vi "2L06-lambda_1D_n1.vi"(0 "OBS/MIF":enum16{"OBS", "MIF"}(ring), 7 "t":dbl[](array[numeric]), 9 "N(t)":u32[](array[numeric]), 11 "error in":errorcluster) -> (4 "Lambda":dbl[](array[numeric]), 15 "error out":errorcluster)   [LabVIEW 2010, in "lv_02.lvlib"]
doc: "Calcul du taux de défaillance à partir de la série t et de la série des effectifs encore en fonctionnement à t :\nObs : précise si les observations sont fournies par rang (n obs) ou par classe (nc classes)\nSi N(t=0) est nul ou non câblé pour les observations de type obs_n, alors n= taille du tableau t"
uses:
  lv_02.lvlib
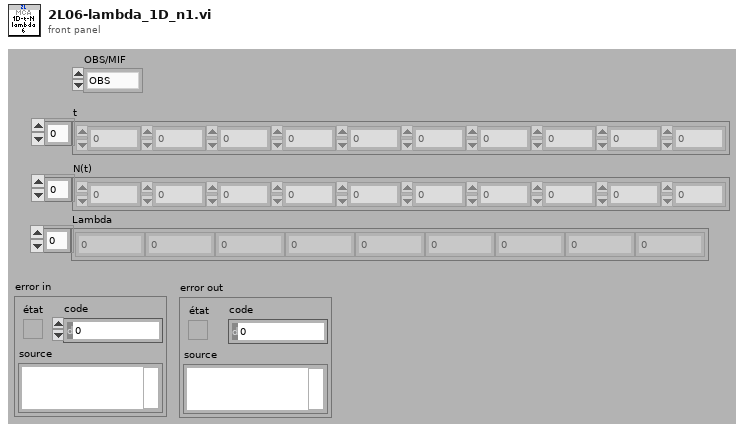
[diagram p1: front panel]
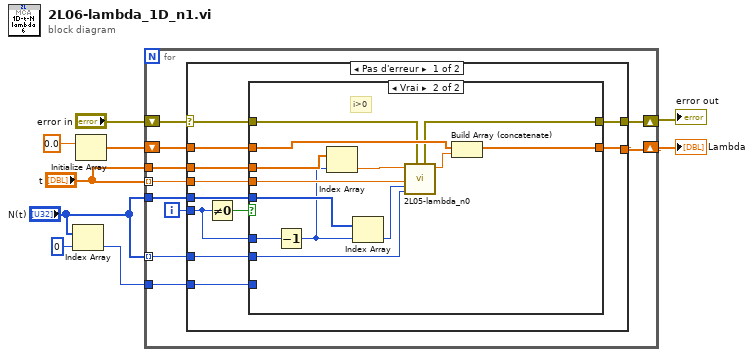
[diagram p0: block diagram]
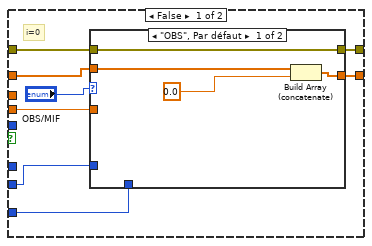
[diagram p2: hidden frame]
diagram:
  n1 = Index Array(array="N(t)", index=0 ("indice")) -> (element=w1:u32)
  n2 = Initialize Array(0.0 ("élément")) -> (w6:dbl[])  [unwired: 1 in]
  n3 = for {
    tunnel: "t" -> [w17]
    tunnel: "t" -> [w19] mode=indexing
    tunnel: "N(t)" -> [w18] mode=indexing
    tunnel: "N(t)" -> [w16]
    shift-right: [w14] -> w4
    shift-left: w6 -> [w15]
    shift-right: [w13] -> w5
    shift-left: "error in" -> [w12]
    tunnel: w1 -> [w10]
    i -> [w11]
    n4 = case shown="Pas d'erreur" w12 {
      selector: w12 -> [w25 w59]
      tunnel: w19 -> [w22 _]
      tunnel: w18 -> [w30 _]
      tunnel: w17 -> [w23 _]
      tunnel: w16 -> [w29 _]
      tunnel: w15 -> [w28 w58]
      tunnel: [w27 w58] -> w14
      tunnel: [w26 w59] -> w13
      tunnel: w11 -> [w21 _]
      tunnel: w10 -> [w20 _]
      frame No Error {
        n5 = Not Equal To 0?(x=w21) -> (x != 0?=w24:bool)
        n6 = case shown="Vrai" w24 {
          tunnel: w29 -> [_ w57]
          tunnel: [w34 w50] -> w27
          tunnel: w30 -> [w38 w56]
          tunnel: w23 -> [_ w55]
          tunnel: w28 -> [w35 w52]
          tunnel: [w33 w49] -> w26
          tunnel: w25 -> [w37 w48]
          tunnel: w22 -> [w36 w47]
          tunnel: w21 -> [_ w46]
          tunnel: w20 -> [w32 _]
          frame False {
            # "i=0"
            n7 = case shown="\"OBS\", Par défaut" "OBS/MIF" {
              tunnel: w38 -> [_ _]
              tunnel: w37 -> [w39 w44]
              tunnel: [w39 w44] -> w33
              tunnel: w36 -> [_ _]
              tunnel: w35 -> [w42 w43]
              tunnel: [w41 w43] -> w34
              tunnel: w32 -> [_ _]
              frame "OBS", Default {
                n8 = Build Array (concatenate)(w42, 0.0 ("lambda")) -> (w41:dbl[])
              }
              frame "MIF" {
              }
            }
          }
          frame True {
            # "i>0"
            n9 = Decrement(x=w46) -> (x-1=w45:i32)
            n10 = Index Array(array=w55, index=w45) -> (element=w54:dbl)
            n11 = Index Array(array=w57, index=w45) -> (element=w53:u32)
            n12 = call "2L05-lambda_n0.vi"("error in (no error)"=w48, "N(tfin)"=w56, "N(tdeb)"=w53, "tfin"=w47, "tdeb"=w54) -> ("lambda"=w51:dbl, "error out"=w49:errorcluster)  [unwired: 3 in]
            n13 = Build Array (concatenate)(w52, w51) -> (w50:dbl[])
          }
        }
      }
      frame Error {
      }
    }
  }
  "Lambda" <- w4
  "error out" <- w5
